vi "JSONObjectToMap.vi"(8 "error in":errorcluster, 10 "Value":variant, 11 "Type":T2(ring)=enum."object") -> (0 "error out":errorcluster, 3 "Map":T1(c390))   [LabVIEW 2020]
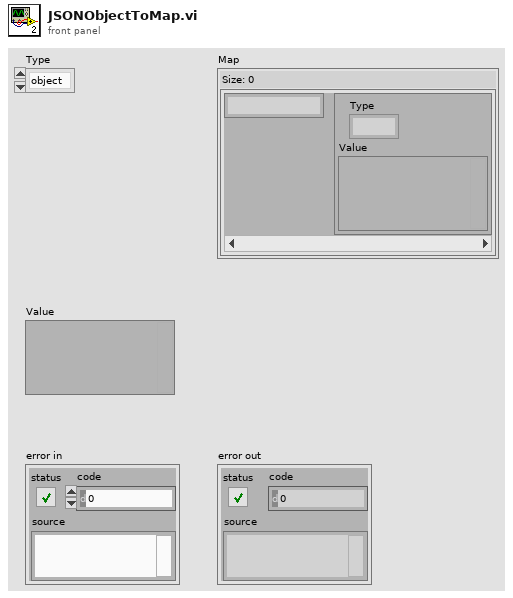
[diagram p1: front panel]
types:
  T1 = map{string, cluster{"Type":enum16{"null", "number", "boolean", "string", "array", "object", ""}, "Value":variant}}
  T2 = enum16{"null", "number", "boolean", "string", "array", "object", ""}
  T3 = cluster{"Key":string, "Value":cluster{"Type":enum16{"null", "number", "boolean", "string", "array", "object", ""}, "Value":variant}}[]
  T4 = cluster{"Type":enum16{"null", "number", "boolean", "string", "array", "object", ""}, "Value":variant}
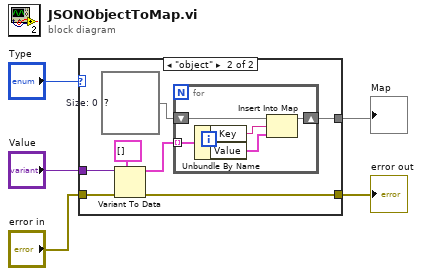
[diagram p0: block diagram]
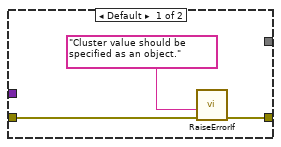
[diagram p2: hidden frame]
diagram:
  n1 = case shown="\"object\"" "Type" {
    tunnel: "Value" -> [_ w14]
    tunnel: [w8 w11] -> w2
    tunnel: "error in" -> [w6 w10]
    tunnel: [_ w9] -> w1
    frame Default {
      n2 = call "RaiseErrorIf.vi"("error in (no error)"=w6, "error message"="Cluster value should be specified as an object." ("error source (\" \")")) -> ("error out"=w8:errorcluster)  [unwired: 9 in]
    }
    frame "object" {
      w13 = T1 {}  # Size: 0
      n3 = Variant To Data(error in=w10, type=T3 [], Variant=w14) -> (data=w12:T3, error out=w11:errorcluster)
      n4 = for {
        shift-right: [w20] -> w9
        shift-left: w13 -> [w19]
        tunnel: w12 -> [w18] mode=indexing
        n5 = Unbundle By Name(w18) -> ("Key"=w17:string, "Value"=w16:T4)
        n6 = Insert Into Map(map in=w19, key=w17, value=w16) -> (map out=w20:T1)  [unwired: 2 out]
      }
    }
  }
  "error out" <- w2
  "Map" <- w1
